vi "Demo.vi"() -> ()   [LabVIEW 2024]
uses:
  <vilib>/picture/3D Picture Control/NI_3D Picture Control.lvlib
panel:
  out "3D Picture":refnum<vi>(3d-picture)
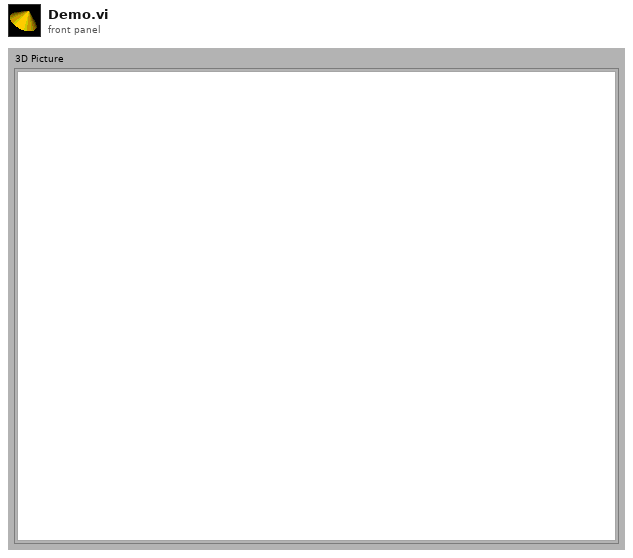
[diagram p1: front panel]
types:
  T1 = cluster{"Text":string, "Color Box":u32, "Alpha":sgl, "Font file":path}
  T2 = cluster{"Height":sgl, "Radius":sgl, "Alpha":sgl, "Color Box":u32, "Detail":sgl}
  T3 = cluster{"Radius":sgl, "Color Box":u32, "Alpha":sgl, "Detail":sgl}
  T4 = cluster{"Height":sgl, "Radius":sgl, "Color Box":u32, "Alpha":sgl, "Detail":sgl}
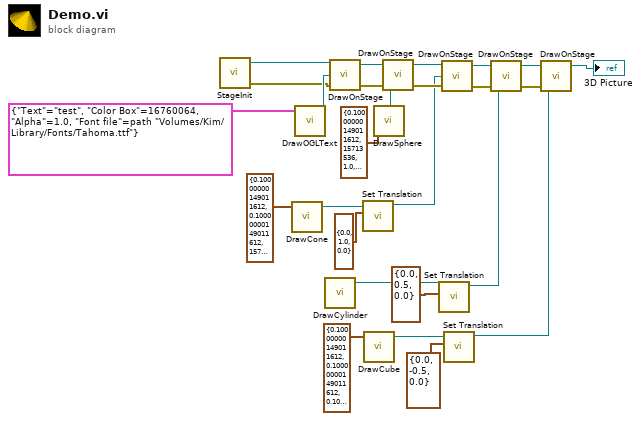
[diagram p0: block diagram]
diagram:
  n1 = call <userlib>:"StageInit.vi"() -> ("error out"=w19:errorcluster, "Stage out"=w20:refnum<vi>)  [unwired: 4 in]
  n2 = call <userlib>:"DrawCone.vi"("Cone"=T4 {"Height"=0.1, "Radius"=0.1, "Color Box"=15713536, "Alpha"=1.0, "Detail"=1.0}) -> ("object out"=w13:refnum<vi>)  [unwired: 5 in, 1 out]
  n3 = call <userlib>:"DrawOGLText.vi"("Text"=T1 {"Text"="test", "Color Box"=16760064, "Alpha"=1.0, "Font file"=path "/Volumes/Kim/Library/Fonts/Tahoma.ttf"}) -> ("object out"=w21:refnum<vi>)  [unwired: 5 in, 1 out]
  n4 = call <userlib>:"DrawCylinder.vi"() -> ("object out"=w24:refnum<vi>)  [unwired: 6 in, 1 out]
  n5 = call <userlib>:"DrawOnStage.vi"("error in"=w19, "object in"=w21, "Stage in"=w20) -> ("error out"=w18:errorcluster, "Stage out"=w17:refnum<vi>)  [unwired: 1 out]
  n6 = call <vilib>:"Set Translation.vi"("Translation"=cluster{"X":sgl, "Y":sgl, "Z":sgl} {"X"=0.0, "Y"=1.0, "Z"=0.0}, "Scene Object"=w13) -> ("Translated Object"=w12:refnum<vi>)  [unwired: 8 in, 1 out]
  n7 = call <userlib>:"DrawCube.vi"("Cube"=T2 {"Height"=0.1, "Radius"=0.1, "Alpha"=0.1, "Color Box"=15713536, "Detail"=1.0} ("Cone")) -> ("object out"=w6:refnum<vi>)  [unwired: 5 in, 1 out]
  n8 = call <userlib>:"DrawSphere.vi"("Sphere"=T3 {"Radius"=0.1, "Color Box"=15713536, "Alpha"=1.0, "Detail"=1.0} ("Cone")) -> ("object out"=w2:refnum<vi>)  [unwired: 5 in, 1 out]
  n9 = call <userlib>:"DrawOnStage.vi"("error in"=w18, "object in"=w2, "Stage in"=w17) -> ("error out"=w16:errorcluster, "Stage out"=w15:refnum<vi>)  [unwired: 1 out]
  n10 = call <vilib>:"Set Translation.vi"("Translation"=cluster{"X":sgl, "Y":sgl, "Z":sgl} {"X"=0.0, "Y"=0.5, "Z"=0.0}, "Scene Object"=w24) -> ("Translated Object"=w9:refnum<vi>)  [unwired: 8 in, 1 out]
  n11 = call <userlib>:"DrawOnStage.vi"("error in"=w16, "object in"=w12, "Stage in"=w15) -> ("error out"=w11:errorcluster, "Stage out"=w10:refnum<vi>)  [unwired: 1 out]
  n12 = call <vilib>:"Set Translation.vi"("Translation"=cluster{"X":sgl, "Y":sgl, "Z":sgl} {"X"=0.0, "Y"=-0.5, "Z"=0.0}, "Scene Object"=w6) -> ("Translated Object"=w5:refnum<vi>)  [unwired: 8 in, 1 out]
  n13 = call <userlib>:"DrawOnStage.vi"("error in"=w11, "object in"=w9, "Stage in"=w10) -> ("error out"=w4:errorcluster, "Stage out"=w8:refnum<vi>)  [unwired: 1 out]
  n14 = call <userlib>:"DrawOnStage.vi"("error in"=w4, "object in"=w5, "Stage in"=w8) -> ("Stage out"=→"3D Picture":refnum<vi>)  [unwired: 2 out]
